vi "Do.vi"(8 "error in (no error)":errorcluster, 10 "Actor in":refnum<class "Actor.lvclass">, 11 "MockNotificationMsg":refnum<class "MockNotificationMsg.lvclass">) -> (0 "error out":errorcluster, 2 "Actor out":refnum<class "Actor.lvclass">)   [LabVIEW 2017, in "MockNotificationMsg.lvclass"]
doc: "(<B>Filename</B>: Actor Framework.lvlib:Message.lvclass:Do.vi)\n\nDefines what a message does when it is received by an actor. Generally, a message instructs an actor to invoke one of its methods. By default, this method does nothing. A child class must override it to define behavior. Create a child class by using the Actor Framework Message Maker dialog box."
uses:
  MockNotificationMsg.lvclass
  C:/Git/composed-transport/Source/Concrete/ActorMessageTransport/Notification Msg/Notification Msg.lvclass
  <vilib>/ActorFramework/Actor/Actor.lvclass
  Source/Concrete/ActorMessageTransport/Notification Msg/Notification Msg.lvclass/Notification Msg.ctl
  MockNotificationMsg.lvclass/MockNotificationMsg.ctl
  Source/Concrete/ActorMessageTransport/Notification Msg/Notification Msg.lvclass
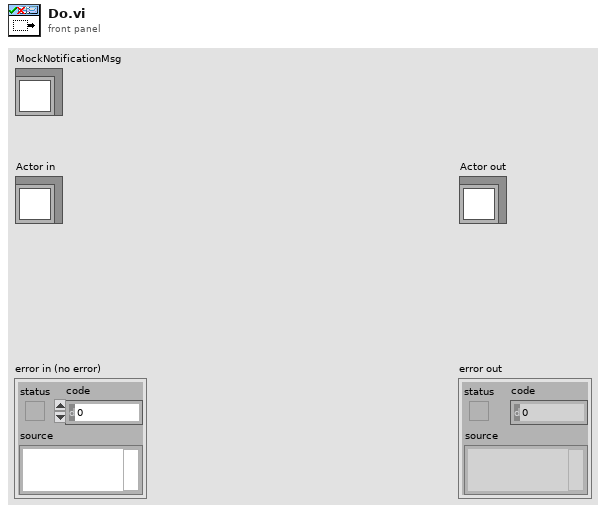
[diagram p1: front panel]
types:
  T1 = cluster{"Datum Name":string, "Value":variant, "Publication Time":timestamp}
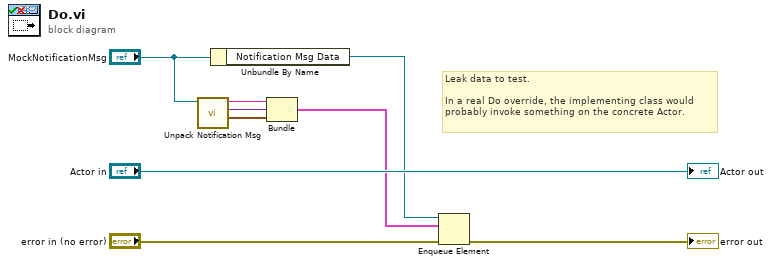
[diagram p0: block diagram]
diagram:
  # "Leak data to test.\n\nIn a real Do override, the implementing class would\nprobably invoke something on the concrete Actor."
  n1 = call "Unpack Notification Msg.vi"("Notification Msg"="MockNotificationMsg") -> ("Publication Time"=w5:timestamp, "Value"=w6:variant, "Datum Name"=w7:string)  [unwired: 8 in]
  n2 = Unbundle By Name("MockNotificationMsg") -> ("Notification Msg Data"=w2:refnum<queue>)
  n3 = Bundle("Datum Name"=w7, "Value"=w6, "Publication Time"=w5) -> (w1:T1)  [unwired: 1 in]
  n4 = Enqueue Element(queue=w2, element=w1, error in (no error)="error in (no error)") -> (error out=→"error out":errorcluster)  [unwired: 1 in, 2 out]
  "Actor out" <- "Actor in"
